vi "Get Variable Container.vi"(8 "error in (no error)":errorcluster, 10 "Type":T2, 11 "TSEngine in":refnum<class "Engine.lvclass">) -> (0 "error out":errorcluster, 2 "VariableContainer":T1, 3 "TSEngine out":refnum<class "Engine.lvclass">)   [LabVIEW 2020, in "HTS.lvlib" / "Engine.lvclass"]
uses:
  Engine.lvclass
  Variable Container Type.ctl
  VariableContainer/Typedefs/Session Handle.ctl
  VariableContainer/VariableContainer.lvclass
  Create VC Event Data.ctl
  Engine.lvclass/Engine.ctl
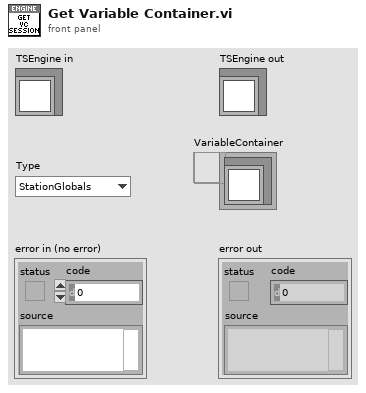
[diagram p1: front panel]
types:
  T1 = typedef "HTS.lvlib/VariableContainer.lvclass/Session Handle.ctl" = refnum<data-value>
  T2 = typedef "HTS.lvlib/Engine.lvclass/Variable Container Type.ctl" = enum16{"StationGlobals", "TemporaryGlobals", "NewPropertyObject"}
  T3 = typedef "HTS.lvlib/Engine.lvclass/Create VC Event Data.ctl" = cluster{"Type":T2, "Notifier":refnum<notifier>}
  T4 = typedef "HTS.lvlib/Engine.lvclass/Events.ctl" = cluster{"Stop Deamon":refnum<user-event>, "Create Variable Container":refnum<user-event>}
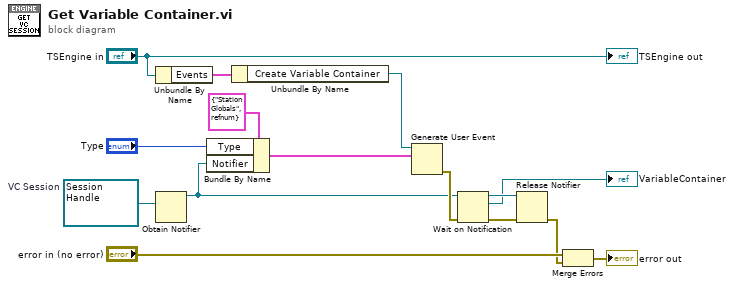
[diagram p0: block diagram]
diagram:
  w14 = T1 refnum  # VC Session
  n1 = Unbundle By Name("TSEngine in") -> ("Events"=w2:T4)
  n2 = Obtain Notifier(notification data type=w14) -> (notifier out=w11:refnum<notifier>)  [unwired: 3 in, 2 out]
  n3 = Bundle By Name(cluster=T3 {"Type"=enum."StationGlobals", "Notifier"=refnum} ("Create Session Event Data"), "Type"="Type", "Notifier"=w11) -> (w10:T3)
  n4 = Unbundle By Name(w2) -> ("Create Variable Container"=w1:refnum<user-event>)
  n5 = Generate User Event(user event=w1, event data cluster=w10) -> (error out=w15:errorcluster)  [unwired: 2 in, 1 out]
  n6 = Wait on Notification(notifier=w11, error in (no error)=w15) -> (notifier out=w7:refnum<notifier>, notification=→"VariableContainer":T1, error out=w6:errorcluster)  [unwired: 2 in, 1 out]
  n7 = Release Notifier(notifier=w7, error in (no error)=w6) -> (error out=w4:errorcluster)  [unwired: 1 in, 2 out]
  n8 = Merge Errors("error in (no error)", w4) -> (→"error out":errorcluster)
  "TSEngine out" <- "TSEngine in"
